vi "Processamento.vi"(0 "Pasta do ensaio":path=path "L:/Documentos/Serviços já concluidos/Tensão residual/Molas Volvo/Dados/Terceiro grupo/Amostra_1_0") -> ()   [LabVIEW 2018]
uses:
  Controles/Infos para processamento.ctl
panel:
  in  "Tab Control":T1(tab)
  in  "R (E2/E1)":dbl=0.1
  in  "Sesc":dbl=600.0 caption="Tensão de escoamento [MPa]"
  in  "Pasta das imagens":path=path "C:/Users/l01481/Documents/Serviços já concluidos/Tensão residual/Molas Volvo/Imagens Volvo"
  in  "Gerar imagens":bool
  out "Uniformidade":cluster{"Array":dbl[], "Array":dbl[]}[](graph)
  out "C plast":cluster{"Resultados":dbl[], dbl[]}[](graph) caption="Correção plasticidade"
  out "Resultados médios":string[][](table)
  out "Resultados":string[][](table)
  out "Infos para processamento":T2={"Diâmetro do furo [mm]"=1.4, "Diâmetro da linha média [mm]"=5.0, "IncF"=0.2, "Módulo de elasticidade [GPa]"=207.0, "Módulo de Poisson"=0.3, "Tipo de roseta utilizada"=enum."Tipo A", "Método de análise"=enum."Simplificado 2008", "Pfinal"=0.3, "Parar auto."=TRUE}
  out "Derivada segunda":cluster{"z":dbl[], "Array":dbl[]}[](graph)
  out "Comparação":cluster{"z":dbl[], "Array":dbl[]}[](graph)
  out "Dados":T3
  # "Programa de processamento para Tensão Residual"
  # "Diâmetro da roseta"
  # "Dados para correção da plasticidade\nModelo Bilinear"
  # "Equações"
  # "P, Q e T são combinações das deformações medidas ponderadas pelos coeficientes da norma"
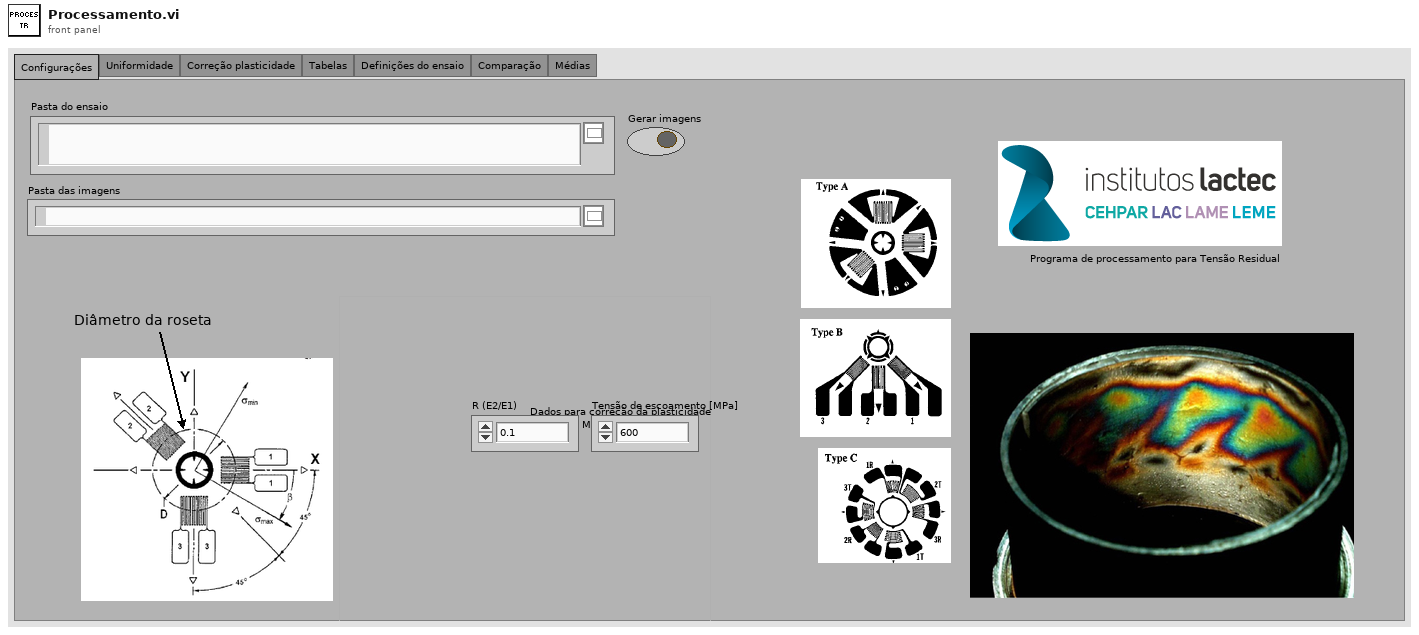
[diagram p1: front panel]
types:
  T1 = enum32{"Configurações", "Uniformidade", "Correção plasticidade", "Tabelas", "Definições do ensaio", "Comparação", "Médias"}
  T2 = typedef "Infos para processamento.ctl" = cluster{"Diâmetro do furo [mm]":dbl, "Diâmetro da linha média [mm]":dbl, "IncF":dbl, "Módulo de elasticidade [GPa]":dbl, "Módulo de Poisson":dbl, "Tipo de roseta utilizada":enum16{"Tipo A", "Tipo B", "Tipo C"}, "Método de análise":enum16{"Não uniforme 2013", "Simplificado 2013", "Simplificado 2008"}, "Pfinal":dbl, "Parar auto.":bool}
  T3 = typedef "Deformações.ctl" = cluster{"def. 1 ":dbl[], "def. 2":dbl[], "def. 3":dbl[], "z":dbl[]}
  T4 = typedef "p,q, t, a e b.ctl" = cluster{"p":dbl[], "q":dbl[], "t":dbl[], "z":dbl[], "a":dbl[], "b":dbl[]}
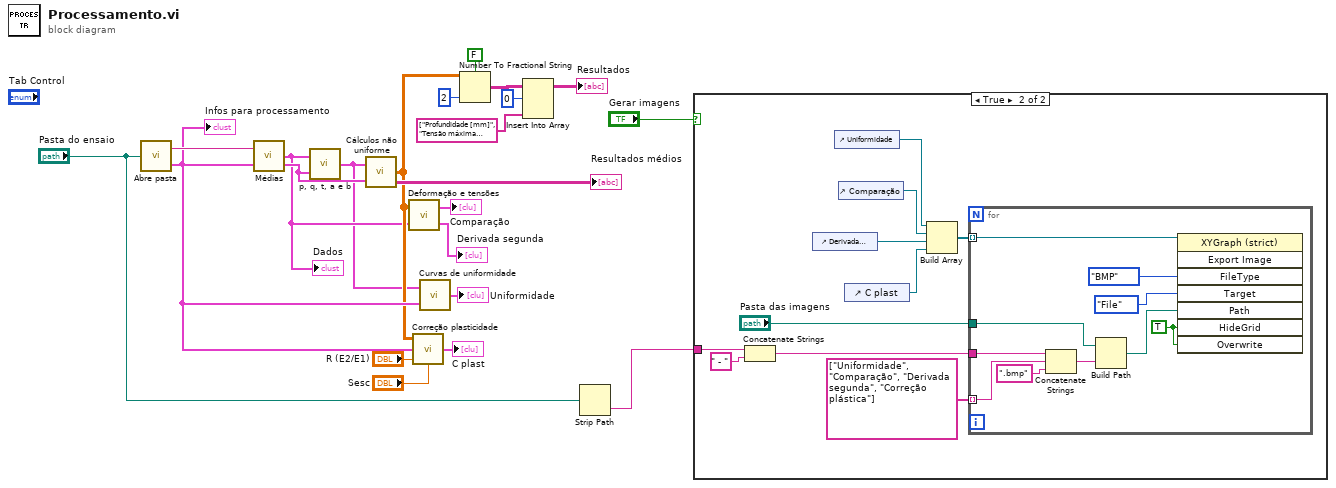
[diagram p0: block diagram]
diagram:
  n1 = call "Abre pasta.vi"("Pasta do ensaio"="Pasta do ensaio") -> ("Dados"=w21:string, "Infos para processamento out"=w20:T2)
  "Infos para processamento" <- w20
  n2 = call "Médias.vi"("Infos para processamento"=w20, "Dados"=w21) -> ("Dados"=w8:T3)
  "Dados" <- w8
  n3 = call "p, q, t, a e b.vi"("Infos para processamento"=w20, "Dados in"=w8) -> ("Dados out"=w2:T4)
  n4 = call "Cálculos não uniforme.vi"("Dados in"=w2, "Infos para processamento in"=w20) -> ("Resultados"=w15:dbl[][], "Resultados médios"=→"Resultados médios":string[][])  [unwired: 1 out]
  n5 = call "Deformação e tensões.vi"("Dados"=w8, "Resultados"=w15) -> ("Derivada"=→"Derivada segunda":cluster{"z":dbl[], "Array":dbl[]}[], "Gráfico"=→"Comparação":cluster{"z":dbl[], "Array":dbl[]}[])
  n6 = call "Correção plasticidade.vi"("Sesc"="Sesc", "R"="R (E2/E1)", "Infos para processamento"=w20, "Resultados"=w15) -> ("Comparação"=→"C plast":cluster{"Resultados":dbl[], dbl[]}[])
  n7 = call "Curvas de uniformidade.vi"("Infos para processamento"=w20, "Dados out"=w2) -> ("Gráficos"=→"Uniformidade":cluster{"Array":dbl[], "Array":dbl[]}[])
  n8 = Number To Fractional String(use system decimal point (T)=FALSE, number=w15, precision (6)=i16 2) -> (F-format string=w12:string[][])  [unwired: 1 in]
  n9 = Insert Into Array(array=w12, index (row)=0, new element=string[] ["Profundidade [mm]", "Tensão máxima [MPa]", "Tensão mínima [MPa]", "Tensão em x [MPa]", "Tensão em y [MPa]", "Tensão cisalhante [MPa]", "Ângulo da tensão máxima [°]", "Tensão de Von Misses [MPa]"] ("new element/subarray")) -> (→"Resultados":string[][])  [unwired: 1 in]
  n10 = Strip Path(path="Pasta do ensaio") -> (name=w16:string)  [unwired: 1 out]
  n11 = case shown="True" "Gerar imagens" {
    tunnel: w16 -> [_ w26]
    frame False {
    }
    frame True {
      n12 = Concatenate Strings(w26, " - " ("string")) -> (w24:string)
      n13 = control-ref of="Derivada segunda"() -> (w29:refnum<vi>)
      n14 = control-ref of="Uniformidade"() -> (w31:refnum<vi>)
      n15 = control-ref of="Comparação"() -> (w30:refnum<vi>)
      n16 = control-ref of="C plast"() -> (w28:refnum<vi>)
      n17 = Build Array(w31, w30, w29, w28) -> (w27:refnum<vi>[])
      n18 = for {
        tunnel: w27 -> [w41] mode=indexing
        tunnel: w24 -> [w38]
        tunnel: string[] ["Uniformidade", "Comparação", "Derivada segunda", "Correção plástica"] -> [w37] mode=indexing
        tunnel: "Pasta das imagens" -> [w34]
        w32 = TRUE ("Hide Grid")
        n19 = Concatenate Strings(w38, w37, ".bmp" ("string")) -> (w35:string)
        n20 = Build Path(base path=w34, name or relative path=w35) -> (appended path=w33:path)
        n21 = invoke class="XYGraph (strict)" method="Export Image"(reference=w41, "FileType"=enum32{"BMP", "EPS", "EMF", "PICT"}."BMP" ("File Type"), "Target"=enum32{"File", "Clipboard"}."File", "Path"=w33, "HideGrid"=w32, "Overwrite"=w32) -> ()  [unwired: 2 in, 8 out]
      }
    }
  }
